vi "PLC_Data_Pallet.vi"(3 "error in (no error)":errorcluster, 4 "condition":string, 5 "Refnum in":T2) -> (0 "error out":errorcluster, 1 "output cluster":T1)   [LabVIEW 2017]
uses:
  <vilib>/ethernetip/ethernetip.llb/ethernetip.ctl
  Control/Main_Data.ctl
  <vilib>/ethernetip/ethernetip.llb/EthernetIPSLC500FileType.ctl
  <vilib>/ethernetip/ethernetip.llb/EthernetIP SLC500 Read Raw.vi
  <vilib>/ethernetip/ethernetip.llb/EthernetIP SLC500 Read Integer.vi
  <vilib>/ethernetip/ethernetip.llb/EthernetIP SLC500 Read Bit.vi
  <vilib>/ethernetip/ethernetip.llb/EthernetIP SLC500 Read Float.vi
  <vilib>/ethernetip/ethernetip.lvlib
panel:
  out "Data":sgl[](array[numeric])
  out "Cycle count":u16
  out "Rejection Count":u16
  out "Alaram":bool[](array[boolean])
  out "OUTPUT":bool[](array[boolean])
  out "Recipe Name":i16
  out "PPH":i16
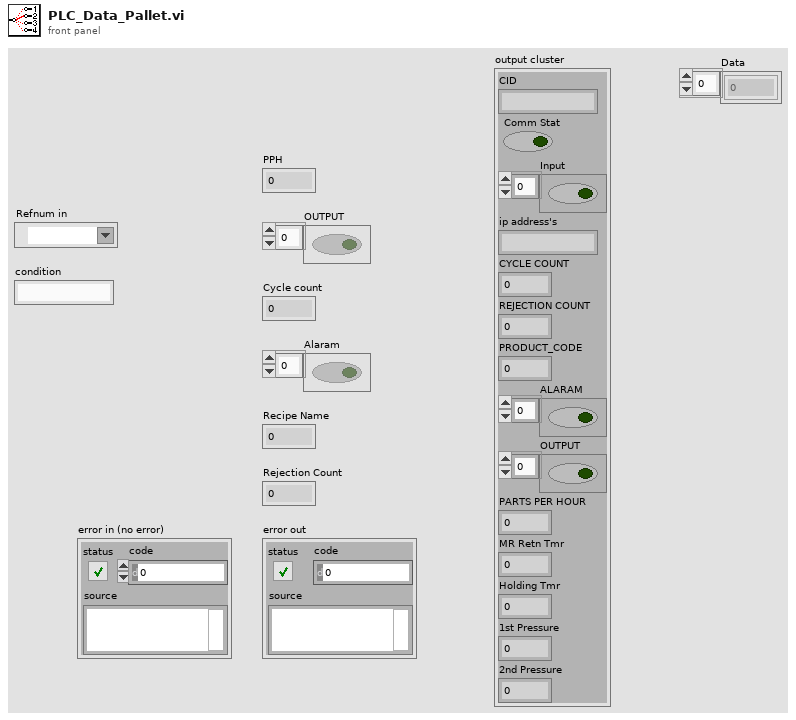
[diagram p1: front panel]
types:
  T1 = typedef "Main_Data.ctl" = cluster{"CID":string, "Comm Stat":bool, "Input":bool[], "ip address's":string, "CYCLE COUNT":u32, "REJECTION COUNT":u32, "PRODUCT_CODE":i16, "ALARAM":bool[], "OUTPUT":bool[], "PARTS PER HOUR":i16, "MR Retn Tmr":dbl, "Holding Tmr":dbl, "1st Pressure":dbl, "2nd Pressure":dbl}
  T2 = typedef "ethernetip.lvlib/ethernetip.ctl" = refnum<k21>
  T3 = typedef "ethernetip.lvlib/EthernetIPSLC500FileType.ctl" = u8
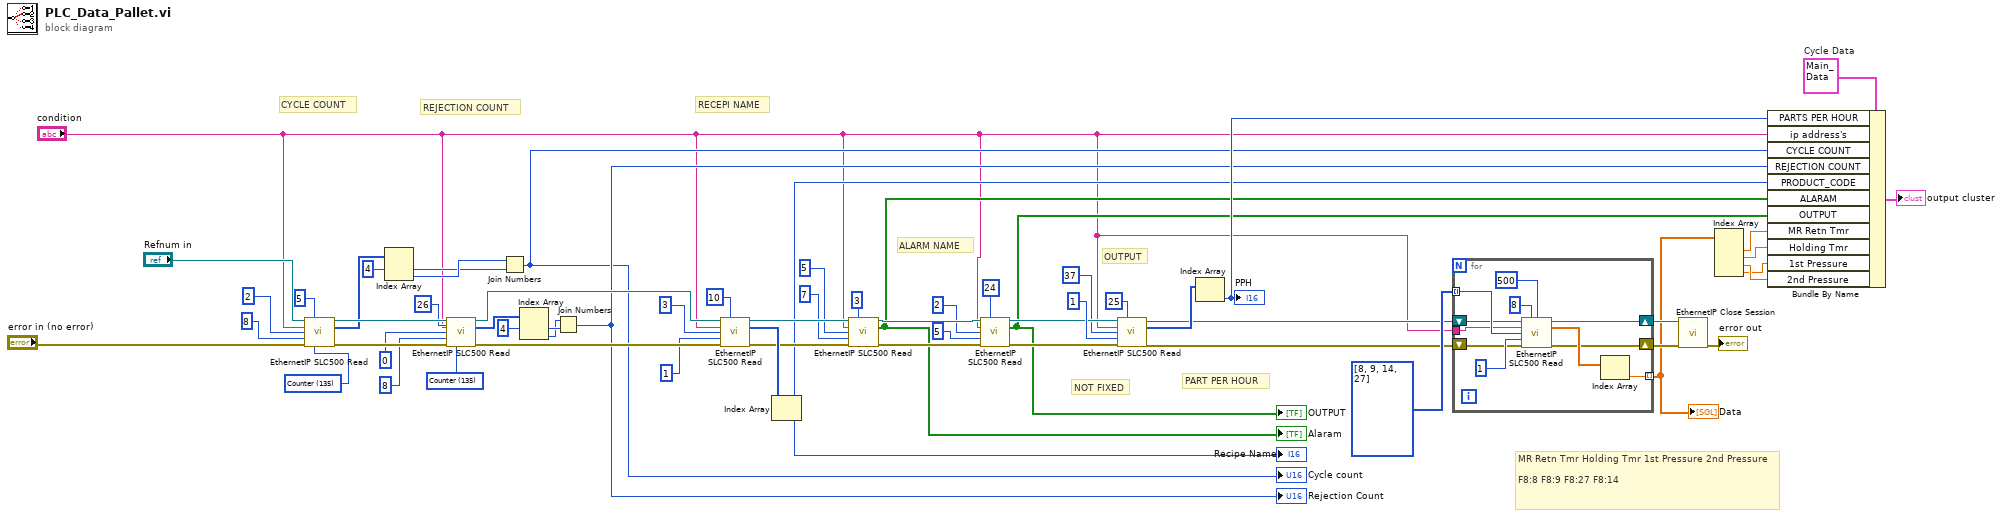
[diagram p0: block diagram]
diagram:
  w19 = T1 {"CID"="", "Comm Stat"=FALSE, "Input"=[FALSE, FALSE, FALSE, FALSE, FALSE], "ip address's"="", "CYCLE COUNT"=0, "REJECTION COUNT"=0, "PRODUCT_CODE"=0, "ALARAM"=[FALSE, FALSE, FALSE, FALSE, FALSE, FALSE, FALSE, FALSE], "OUTPUT"=[FALSE, FALSE, FALSE, FALSE, FALSE], "PARTS PER HOUR"=0, "MR Retn Tmr"=0.0, "Holding Tmr"=0.0, "1st Pressure"=0.0, "2nd Pressure"=0.0}  # Cycle Data
  w32 = T3 135 items=["Status"=132, "Bit"=133, "Timer"=134, "Counter"=135, "Control"=136, "Integer"=137, "Float"=138, "Output"=139, "Input"=140, "String"=141, "ASCII"=142] ("File Type")
  w22 = T3 135 items=["Status"=132, "Bit"=133, "Timer"=134, "Counter"=135, "Control"=136, "Integer"=137, "Float"=138, "Output"=139, "Input"=140, "String"=141, "ASCII"=142] ("File Type")
  # "MR Retn Tmr\tHolding Tmr\t1st Pressure\t2nd Pressure\n\t\t\t\nF8:8\tF8:9\tF8:27\tF8:14"
  # "NOT FIXED"
  # "PART PER HOUR"
  # "OUTPUT"
  # "ALARM NAME"
  # "RECEPI NAME"
  # "REJECTION COUNT"
  # "CYCLE COUNT"
  n1 = call-poly <vilib>:"EthernetIP SLC500 Read.vi"("Session in"="Refnum in", "File Number"=u16 5, "Network Path"="condition", "Element Number"=u16 2, "Number of Bytes"=u32 8, "error in"="error in (no error)", "File Type"=w22) -> ("Session out"=w51:T2, "Data"=w24:u8[], "error out"=w34:errorcluster)  [unwired: 6 in]
  n2 = Index Array(array=w24, index #1=4 ("index")) -> (element #1=w25:u8, element #2=w26:u8)  [unwired: 1 in]
  n3 = call-poly <vilib>:"EthernetIP SLC500 Read.vi"("Session in"=w51, "File Number"=u16 26, "Network Path"="condition", "Element Number"=u16 0, "Number of Bytes"=u32 8, "error in"=w34, "File Type"=w32) -> ("Session out"=w52:T2, "Data"=w29:u8[], "error out"=w45:errorcluster)  [unwired: 6 in]
  n4 = Join Numbers(hi=w26, lo=w25) -> ((hi.lo)=w13:u16)
  "Cycle count" <- w13
  n5 = Index Array(array=w29, index #1=4 ("index")) -> (element #1=w28:u8, element #2=w27:u8)  [unwired: 1 in]
  n6 = Join Numbers(hi=w27, lo=w28) -> ((hi.lo)=w14:u16)
  "Rejection Count" <- w14
  n7 = call-poly <vilib>:"EthernetIP SLC500 Read.vi"("Session in"=w52, "File Number"=u16 10, "Network Path"="condition", "Element Number"=u16 3, "Number of Elements"=u32 1 ("Number of Bytes"), "error in"=w45) -> ("Session out"=w53:T2, "Data"=w56:i16[], "error out"=w46:errorcluster)  [unwired: 7 in]
  n8 = Index Array(array=w56) -> (element=w15:i16)  [unwired: 1 in]
  "Recipe Name" <- w15
  n9 = call-poly <vilib>:"EthernetIP SLC500 Read.vi"("Session in"=w53, "File Number"=u16 3, "Network Path"="condition", "Element Number"=u16 5, "Number of Bits"=u32 7 ("Number of Bytes"), "error in"=w46) -> ("Session out"=w54:T2, "Data"=w16:bool[], "error out"=w43:errorcluster)  [unwired: 7 in]
  "Alaram" <- w16
  n10 = call-poly <vilib>:"EthernetIP SLC500 Read.vi"("Session in"=w54, "File Number"=u16 24, "Network Path"="condition", "Element Number"=u16 2, "Number of Bits"=u32 5 ("Number of Bytes"), "error in"=w43) -> ("Session out"=w61:T2, "Data"=w17:bool[], "error out"=w60:errorcluster)  [unwired: 7 in]
  "OUTPUT" <- w17
  n11 = call-poly <vilib>:"EthernetIP SLC500 Read.vi"("Session in"=w61, "File Number"=u16 25, "Network Path"="condition", "Element Number"=u16 37, "Number of Elements"=u32 1, "error in"=w60) -> ("Session out"=w8:T2, "Data"=w57:i16[], "error out"=w9:errorcluster)  [unwired: 7 in]
  n12 = Index Array(array=w57) -> (element=w18:i16)  [unwired: 1 in]
  "PPH" <- w18
  n13 = for {
    tunnel: [w68] -> w5 mode=indexing
    tunnel: u16[] [8, 9, 14, 27] ("Element Number") -> [w70] mode=indexing
    shift-right: [w67] -> w10
    shift-left: w9 -> [w66]
    tunnel: "condition" -> [w64]
    shift-right: [w63] -> w6
    shift-left: w8 -> [w65]
    n14 = call-poly <vilib>:"EthernetIP SLC500 Read.vi"("Session in"=w65, "File Number"=u16 8, "Timeout (ms)"=500, "Network Path"=w64, "Element Number"=w70, "Number of Elements"=u32 1, "error in"=w66) -> ("Session out"=w63:T2, "Data"=w69:sgl[], "error out"=w67:errorcluster)  [unwired: 6 in]
    n15 = Index Array(array=w69) -> (element=w68:sgl)  [unwired: 1 in]
  }
  "Data" <- w5
  n16 = call <vilib>:"EthernetIP Close Session.vi"("error in"=w10, "Session in"=w6) -> ("error out"=→"error out":errorcluster)  [unwired: 9 in]
  n17 = Index Array(array=w5) -> (element #1=w4:sgl, element #2=w3:sgl, element #3=w2:sgl, element #4=w1:sgl)  [unwired: 4 in]
  n18 = Bundle By Name(cluster=w19, "PARTS PER HOUR"=w18, "ip address's"="condition", "CYCLE COUNT"=w13, "REJECTION COUNT"=w14, "PRODUCT_CODE"=w15, "ALARAM"=w16, "OUTPUT"=w17, "MR Retn Tmr"=w4, "Holding Tmr"=w3, "1st Pressure"=w1, "2nd Pressure"=w2) -> (→"output cluster":T1)
